vi "PH_Sixpack.set i Attri.vi"(2 "error in (no error)":errorcluster, 3 "Instance Name":string) -> (0 "error out":errorcluster, 1 "i Attributes":T2={"Information"={"SixPack ID(0)"=0, "BaudRate(19200)"=19200, "COM Port"=enum."COM1", "HANDLE"=0}, "Serial Number"=-1.0, "Firmwareversion"=-1.0, "Axes"=[], "Status"=enum."None", "Axis to do a RefSearch"=-1, "GUI Refs"={"Information"=refnum, "Serial Number"=refnum, "Firmwareversion"=refnum, "Status"=refnum, "Axis to do a RefSearch"=refnum, "Axes Configuration (Sixpack)"=refnum, "Inputs"=refnum, "PeriodicInterval [ms]"=refnum}, "Constructor finished"=FALSE, "Ignore Error"=FALSE} {"Axes"."Config"."Axis Parameter"."Poslimit (6400)" step=1; "Axes"."Config"."Ref Search Parameter"."DebouncingTime (22ms)" format="%.0x"; "Axes"."Config"."I max (50%)" min=0.0 max=100.0})   [LabVIEW 2014, in "PH_Sixpack.lvlib"]
uses:
  PH_Sixpack.lvlib
  PH_Sixpack.i attribute.ctl
  PH_Sixpack.Axis Cluster.ctl
  PH_Sixpack.Axis Configuration.ctl
  instr.lib/SixPack/PackDLL/VmaxAmax.ctl
  instr.lib/SixPack/PackDLL/PeakCurrent.ctl
  instr.lib/SixPack/PackDLL/VStartVmin.ctl
  instr.lib/SixPack/PackDLL/Ref Search Parameter.ctl
  instr.lib/SixPack/PackDLL/Stopswitch Limits.ctl
  instr.lib/SixPack/PackDLL/Motor Parameter.ctl
  instr.lib/SixPack/PackDLL/MotorParameter_P5.ctl
  instr.lib/SixPack/PackDLL/MotorParameter_P6.ctl
  instr.lib/SixPack/PackDLL/Current Control.ctl
  instr.lib/SixPack/PackDLL/Current.ctl
  PH_Sixpack.Status.ctl
  instr.lib/SixPack/Sixpack - Driver.lvlib
panel:
  in  "COM Port":T1(ring)=enum."COM2"
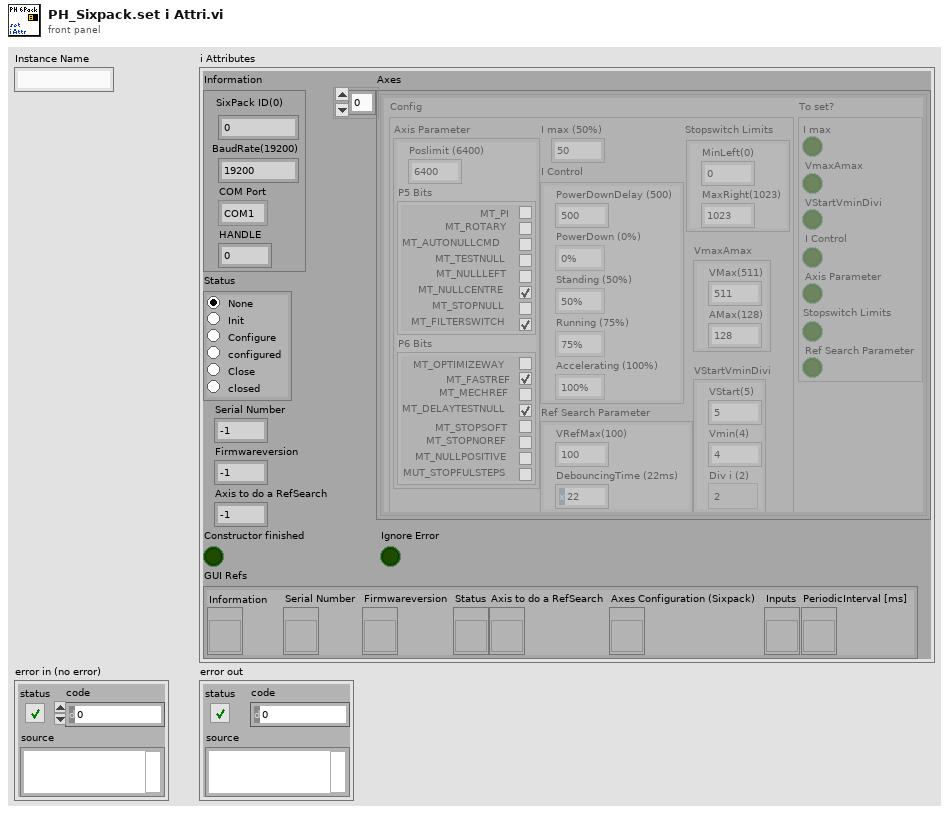
[diagram p1: front panel]
types:
  T1 = enum32{"COM1", "COM2", "COM3", "COM4", "COM5", "COM6", "COM7", "COM8", "COM9"}
  T2 = typedef "PH_Sixpack.lvlib/PH_Sixpack.i attribute.ctl" = cluster{"Information":cluster{"SixPack ID(0)":u16, "BaudRate(19200)":u16, "COM Port":enum32{"COM1", "COM2", "COM3", "COM4", "COM5", "COM6", "COM7", "COM8", "COM9"}, "HANDLE":i32}, "Serial Number":dbl, "Firmwareversion":dbl, "Axes":T3[], "Status":T15, "Axis to do a RefSearch":i32, "GUI Refs":cluster{"Information":refnum<vi>, "Serial Number":refnum<vi>, "Firmwareversion":refnum<vi>, "Status":refnum<vi>, "Axis to do a RefSearch":refnum<vi>, "Axes Configuration (Sixpack)":refnum<vi>, "Inputs":refnum<vi>, "PeriodicInterval [ms]":refnum<vi>}, "Constructor finished":bool, "Ignore Error":bool}
  T3 = typedef "PH_Sixpack.lvlib/PH_Sixpack.Axis Cluster.ctl" = cluster{"Config":T4, "To set?":cluster{"VmaxAmax":bool, "I max":bool, "VStartVminDivi":bool, "Ref Search Parameter":bool, "Stopswitch Limits":bool, "Axis Parameter":bool, "I Control":bool}}
  T4 = typedef "PH_Sixpack.lvlib/PH_Sixpack.Axis Configuration.ctl" = cluster{"VmaxAmax":T5, "I max (50%)":T6, "VStartVminDivi":T7, "Ref Search Parameter":T8, "Stopswitch Limits":T9, "Axis Parameter":T10, "I Control":T13}
  T5 = typedef "Sixpack - Driver.lvlib/VmaxAmax.ctl" = cluster{"VMax(511)":u16, "AMax(128)":u16}
  T6 = typedef "Sixpack - Driver.lvlib/PeakCurrent.ctl" = dbl
  T7 = typedef "Sixpack - Driver.lvlib/VStartVmin.ctl" = cluster{"VStart(5)":u16, "Vmin(4)":u16, "Div i (2)":enum8{"0", "1", "2", "3"}}
  T8 = typedef "Sixpack - Driver.lvlib/Ref Search Parameter.ctl" = cluster{"VRefMax(100)":u16, "DebouncingTime (22ms)":u8}
  T9 = typedef "Sixpack - Driver.lvlib/Stopswitch Limits.ctl" = cluster{"MinLeft(0)":u16, "MaxRight(1023)":u16}
  T10 = typedef "Sixpack - Driver.lvlib/Motor Parameter.ctl" = cluster{"Poslimit (6400)":u32, "P5 Bits":T11, "P6 Bits":T12}
  T11 = typedef "Sixpack - Driver.lvlib/MotorParameter_P5.ctl" = cluster{"MT_PI":bool, "MT_ROTARY":bool, "MT_AUTONULLCMD":bool, "MT_TESTNULL":bool, "MT_NULLLEFT":bool, "MT_NULLCENTRE":bool, "MT_STOPNULL":bool, "MT_FILTERSWITCH":bool}
  T12 = typedef "Sixpack - Driver.lvlib/MotorParameter_P6.ctl" = cluster{"MT_OPTIMIZEWAY":bool, "MT_FASTREF":bool, "MT_MECHREF":bool, "MT_DELAYTESTNULL":bool, "MT_STOPSOFT":bool, "MT_STOPNOREF":bool, "MT_NULLPOSITIVE":bool, "MUT_STOPFULSTEPS":bool}
  T13 = typedef "Sixpack - Driver.lvlib/Current Control.ctl" = cluster{"PowerDownDelay (500)":u16, "PowerDown (0%)":T14, "Standing (50%)":T14, "Running (75%)":T14, "Accelerating (100%)":T14}
  T14 = typedef "Sixpack - Driver.lvlib/Current.ctl" = enum8{"100%", "75%", "50%", "38%", "25%", "19%", "13%", "9%", "0%"}
  T15 = typedef "PH_Sixpack.lvlib/PH_Sixpack.Status.ctl" = enum32{"None", "Init", "Configure", "configured", "Close", "closed"}
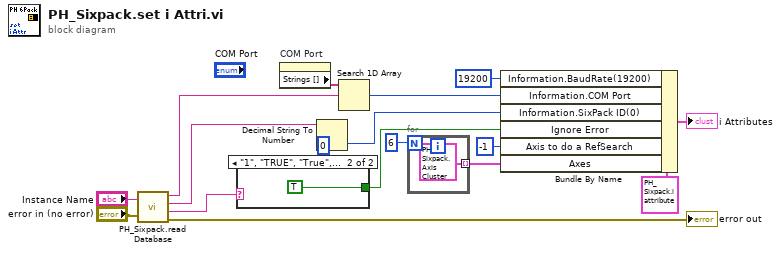
[diagram p0: block diagram]
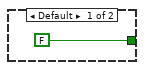
[diagram p2: hidden frame]
diagram:
  n1 = call "PH_Sixpack.read Database.vi"("DB Entry to read"="Instance Name", "error in (no error)"="error in (no error)") -> ("COM Port"=w4:string, "SixPack ID"=w2:string, "Ignore Error"=w6:string, "error out"=→"error out":errorcluster)
  n2 = case shown="\"1\", \"TRUE\", \"True\", \"ja\", \"jawoll\", \"true\"" w6 {
    tunnel: [FALSE TRUE] -> w10
    frame Default {
    }
    frame "1", "TRUE", "True", "ja", "jawoll", "true" {
    }
  }
  n3 = property on="COM Port" class="Enum (strict)"() -> ("Strings []"=w9:string[])  [unwired: 2 in, 2 out]
  n4 = Decimal String To Number(string=w2, default (0L)=u16 0 ("default (0 I32)")) -> (number=w1:u16)  [unwired: 1 in, 1 out]
  n5 = Search 1D Array(1D array=w9, element=w4) -> (index of element=w3:i32)  [unwired: 1 in]
  n6 = for {
    N: 6 -> [_]
    tunnel: [T3 {"Config"={"VmaxAmax"={"VMax(511)"=511, "AMax(128)"=128}, "I max (50%)"=50.0, "VStartVminDivi"={"VStart(5)"=5, "Vmin(4)"=4, "Div i (2)"=enum."2"}, "Ref Search Parameter"={"VRefMax(100)"=100, "DebouncingTime (22ms)"=34}, "Stopswitch Limits"={"MinLeft(0)"=0, "MaxRight(1023)"=1023}, "Axis Parameter"={"Poslimit (6400)"=6400, "P5 Bits"={"MT_PI"=FALSE, "MT_ROTARY"=FALSE, "MT_AUTONULLCMD"=FALSE, "MT_TESTNULL"=FALSE, "MT_NULLLEFT"=FALSE, "MT_NULLCENTRE"=TRUE, "MT_STOPNULL"=FALSE, "MT_FILTERSWITCH"=TRUE}, "P6 Bits"={"MT_OPTIMIZEWAY"=FALSE, "MT_FASTREF"=TRUE, "MT_MECHREF"=FALSE, "MT_DELAYTESTNULL"=TRUE, "MT_STOPSOFT"=FALSE, "MT_STOPNOREF"=FALSE, "MT_NULLPOSITIVE"=FALSE, "MUT_STOPFULSTEPS"=FALSE}}, "I Control"={"PowerDownDelay (500)"=500, "PowerDown (0%)"=enum."0%", "Standing (50%)"=enum."50%", "Running (75%)"=enum."75%", "Accelerating (100%)"=enum."100%"}}, "To set?"={"VmaxAmax"=FALSE, "I max"=FALSE, "VStartVminDivi"=FALSE, "Ref Search Parameter"=FALSE, "Stopswitch Limits"=FALSE, "Axis Parameter"=FALSE, "I Control"=FALSE}} ("motor")] -> w17 mode=indexing
  }
  n7 = Bundle By Name(cluster=T2 {"Information"={"SixPack ID(0)"=0, "BaudRate(19200)"=0, "COM Port"=enum."COM1", "HANDLE"=0}, "Serial Number"=0.0, "Firmwareversion"=0.0, "Axes"=[], "Status"=enum."None", "Axis to do a RefSearch"=0, "GUI Refs"={"Information"=refnum, "Serial Number"=refnum, "Firmwareversion"=refnum, "Status"=refnum, "Axis to do a RefSearch"=refnum, "Axes Configuration (Sixpack)"=refnum, "Inputs"=refnum, "PeriodicInterval [ms]"=refnum}, "Constructor finished"=FALSE, "Ignore Error"=FALSE} ("CLASS.i attribute"), "Information.BaudRate(19200)"=u16 19200, "Information.COM Port"=w3, "Information.SixPack ID(0)"=w1, "Ignore Error"=w10, "Axis to do a RefSearch"=-1, "Axes"=w17) -> (→"i Attributes":T2)
